vi "Pot Value To Angle.vi"(0 "potOutput":dbl, 1 "Offset Constant (b)":dbl, 2 "right most angle":dbl, 3 "left most angle":dbl, 4 "right most pot val":dbl=1.0, 5 "left most pot val":dbl=-1.0) -> (7 "angle":dbl)   [LabVIEW 2016]
panel:
  out "Scaling Value (m)":dbl
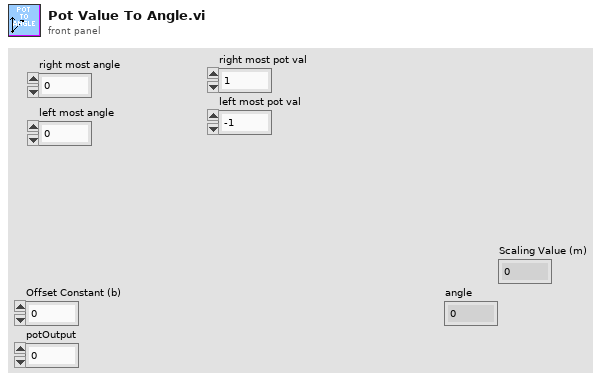
[diagram p1: front panel]
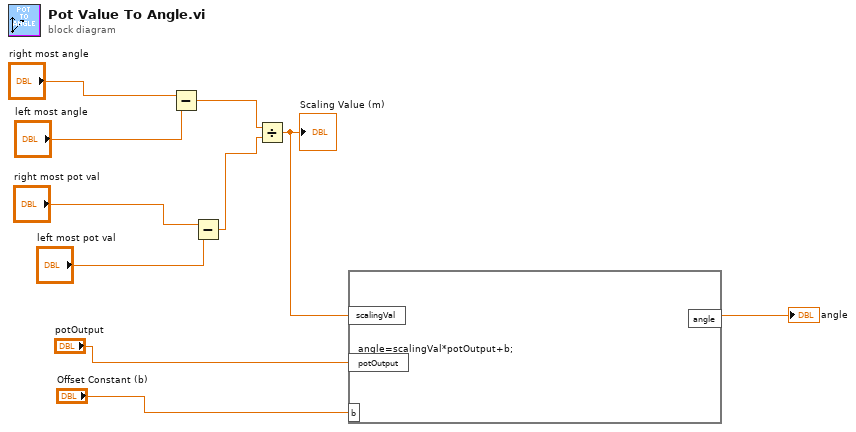
[diagram p0: block diagram]
diagram:
  n1 = Subtract(x="right most angle", y="left most angle") -> (x-y=w4:dbl)
  n2 = Subtract(x="right most pot val", y="left most pot val") -> (x-y=w3:dbl)
  n3 = Divide(x=w4, y=w3) -> (x/y=w2:dbl)
  "Scaling Value (m)" <- w2
  n4 = formula code="angle=scalingVal*potOutput+b;"("scalingVal"=w2, "potOutput"="potOutput", "b"="Offset Constant (b)") -> ("angle"=→"angle":dbl)
